vi "clearpath_set_safety_system.vi"(0 "ClearpathComm":T1, 1 "Set Stop Flag":bool) -> ()   [LabVIEW 2012, in "clearpath_interface.lvlib"]
doc: "Formats a Set Safety System command (0x10) to set or release the software controlled emergency stop. Uses the onboard Clearpath library to perform the actual message formatting."
uses:
  clearpath_interface.lvlib
  cwrap_crio.dll
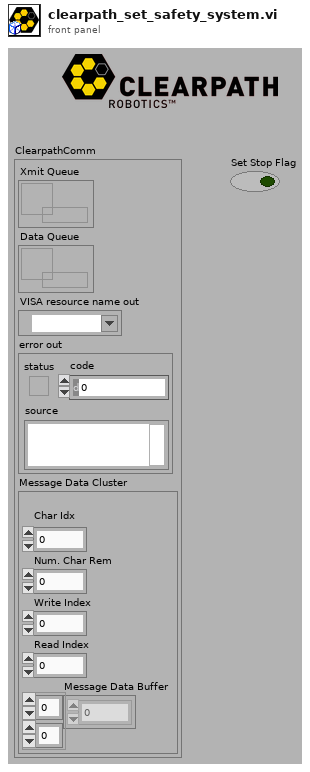
[diagram p1: front panel]
types:
  T1 = cluster{"Xmit Queue":refnum<queue>, "Data Queue":refnum<queue>, "VISA resource name out":refnum<visa-resource-name>, "error out":errorcluster, "Message Data Cluster":cluster{"\nChar Idx":u8, "Num. Char Rem":u8, "Write Index":u8, "Read Index":u8, "Message Data Buffer":u8[][]}}
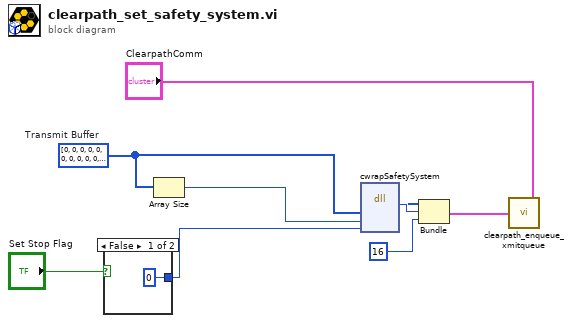
[diagram p0: block diagram]
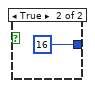
[diagram p2: hidden frame]
diagram:
  w6 = u8[] [0, 0, 0, 0, 0, 0, 0, 0, 0, 0, 0, 0, 0, 0, 0, 0, 0, 0, 0, 0, 0, 0, 0, 0, 0, 0, 0, 0, 0, 0, 1, 0, 0, 0, 5]  # Transmit Buffer
  n1 = case shown="False" "Set Stop Flag" {
    tunnel: [0 16] -> w4
    frame False {
    }
    frame True {
    }
  }
  n2 = Array Size(array=w6) -> (size(s)=w7:i32)
  n3 = dll-call lib="C:/Users/tebbeam/Documents/GitHub/IGVC-2013/Code/Project 1.0/Motors/Husky/cwrap_cRIO.*" fn="cwrapSafetySystem"("buf"=w6, "buf_size"=w7, "flags"=w4) -> ("return type"=w9:i32, "buf"=w8:u8[])  [unwired: 5 in, 2 out]
  n4 = Bundle("buf"=w8, "return type"=w9, 16) -> (w1:cluster{"buf":u8[], "return type":i32, i32})  [unwired: 1 in]
  n5 = call "clearpath_enqueue_xmitqueue.vi"("ClearpathComm"="ClearpathComm", "Cluster"=w1) -> ()
